vi "LVITX Remove Illegal Characters from Wavename.vi"(1 "Wavenames":string) -> (0 "Wavenames with Illegal Characters removed":string)   [LabVIEW 2011]
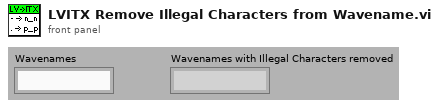
[diagram p1: front panel]
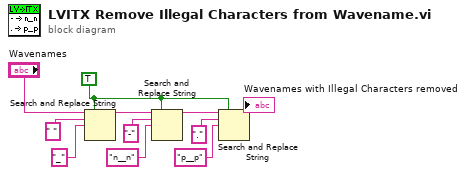
[diagram p0: block diagram]
diagram:
  w9 = TRUE ("replace all? (F)")
  n1 = Search and Replace String(replace all?=w9, input string="Wavenames", search string=" ", replace string="_" ("replace string (\"\")")) -> (result string=w7:string)  [unwired: 4 in, 3 out]
  n2 = Search and Replace String(replace all?=w9, input string=w7, search string="-", replace string="n__n" ("replace string (\"\")")) -> (result string=w4:string)  [unwired: 4 in, 3 out]
  n3 = Search and Replace String(replace all?=w9, input string=w4, search string=".", replace string="p__p" ("replace string (\"\")")) -> (result string=→"Wavenames with Illegal Characters removed":string)  [unwired: 4 in, 3 out]
